vi "Example.vi"(8 "error in (no error)":errorcluster, 10 "Output Voltage":dbl format="%.4f", 11 "VISA name":refnum<visa-resource-name>="GPIB::5::INSTR") -> (0 "error out":errorcluster, 2 "Measured Voltage":dbl format="%.4f")   [LabVIEW 2020, in "Low Level PSU.lvlib"]
uses:
  Low Level PSU.lvlib
  Low Level PSU.lvclass
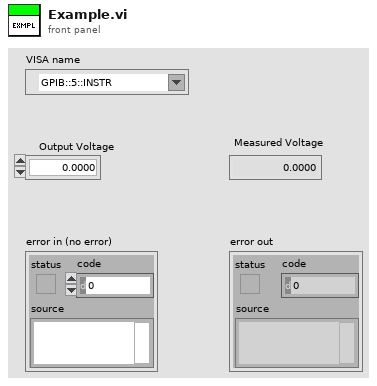
[diagram p1: front panel]
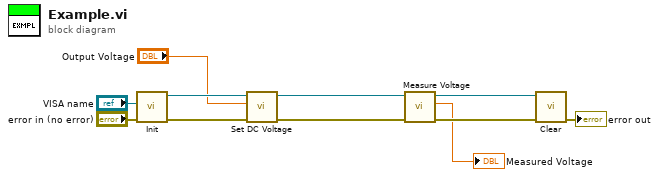
[diagram p0: block diagram]
diagram:
  n1 = call "Init.vi"("error in (no error)"="error in (no error)", "VISA name"="VISA name") -> ("error out"=w10:errorcluster, "Low Level PSU Out"=w11:refnum<class "Low Level PSU.lvclass">)  [unwired: 8 in]
  n2 = call "Set DC Voltage.vi"("error in (no error)"=w10, "Volt"="Output Voltage", "Low Level PSU in"=w11) -> ("error out"=w8:errorcluster, "Low Level PSU out"=w9:refnum<class "Low Level PSU.lvclass">)  [unwired: 7 in]
  n3 = call "Measure Voltage.vi"("error in (no error)"=w8, "Low Level PSU In"=w9) -> ("error out"=w6:errorcluster, "Output Voltage"=→"Measured Voltage":dbl, "Low Level PSU Out"=w7:refnum<class "Low Level PSU.lvclass">)  [unwired: 7 in]
  n4 = call "Clear.vi"("error in (no error)"=w6, "Low Level PSU In"=w7) -> ("error out"=→"error out":errorcluster)  [unwired: 8 in, 1 out]
